vi "MotionCharacterization.vi"() -> ()   [LabVIEW 2011]
panel:
  out "Avg. Motion Time":dbl(knob) scale=0.0..100.0
  out "Joints":T1(graph)
  out "Cartesian":T1(graph)
  out "Coordinates sent to robot:":string
  out "Data Valid?":bool
  out "Motion Timing":u32(graph)
  in  "stop":bool
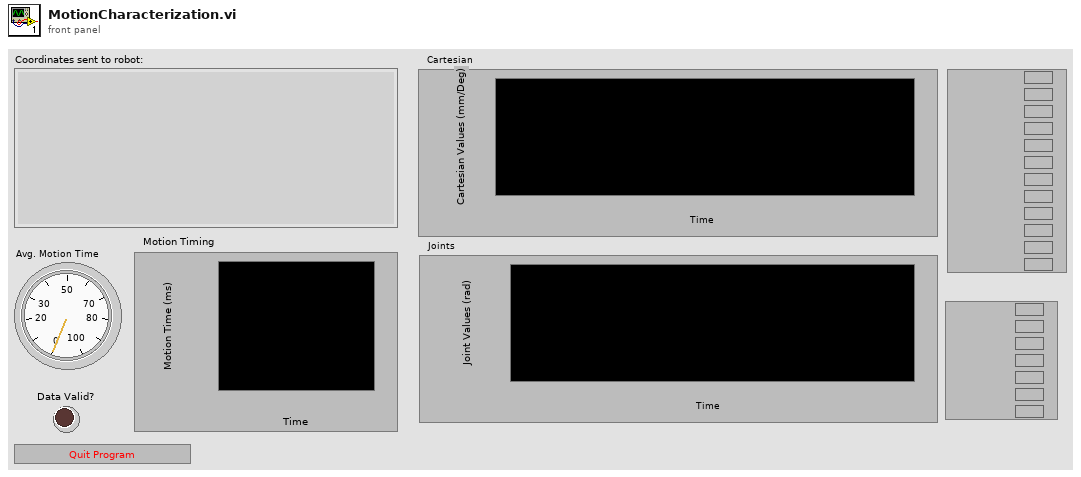
[diagram p1: front panel]
types:
  T1 = cluster{"Data Out[0]":dbl, "Data Out[1]":dbl, "Data Out[2]":dbl, "Data Out[3]":dbl, "Data Out[4]":dbl, "Data Out[5]":dbl, "Data Out[6]":dbl, "Data Out[7]":dbl, "Data Out[8]":dbl}
  T2 = enum16{"Standard", "Buffered", "CRLF", "Immediate"}
  T3 = cluster{"[0]":dbl, "[1]":dbl, "[2]":dbl, "[3]":dbl, "[4]":dbl, "[5]":dbl, "[6]":dbl, "[7]":dbl, "[8]":dbl}
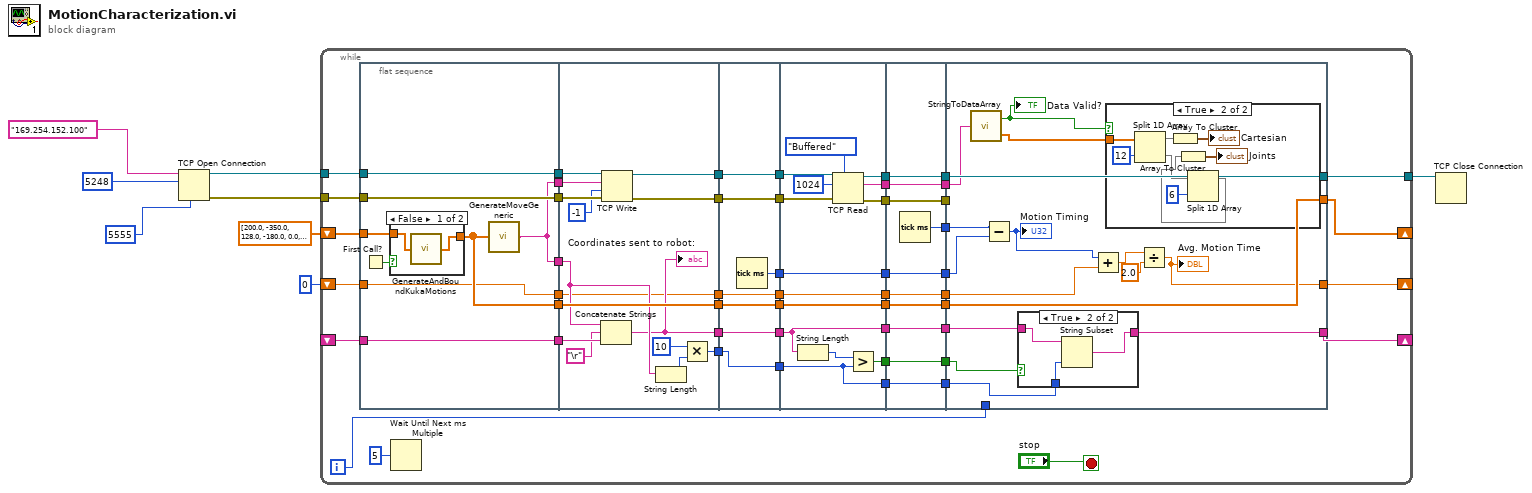
[diagram p0: block diagram]
diagram:
  n1 = TCP Open Connection(address="169.254.152.100", remote port or service name=u16 5248, local port=u16 5555 ("local port (0)")) -> (connection ID=w8:refnum<k5>, error out=w6:errorcluster)  [unwired: 2 in]
  n2 = while {
    tunnel: w8 -> [w58]
    tunnel: [w57] -> w7
    tunnel: w6 -> [w56]
    shift-right: [w37] -> _
    shift-left: dbl[] [200.0, -350.0, 128.0, -180.0, 0.0, 90.0] ("Output Array") -> [w36]
    shift-right: [w26] -> _
    shift-left: _ -> [w28]
    shift-right: [w15] -> _
    shift-left: u32 0 -> [w9]
    i -> [w30]
    stop <- "stop" stop-if-true
    n3 = flat-sequence {
      tunnel: w56 -> [w66]
      tunnel: w58 -> [w67]
      tunnel: [w67] -> w54
      tunnel: [w66] -> w53
      tunnel: [w62] -> w48
      tunnel: w36 -> [w64]
      tunnel: [w63] -> w31
      tunnel: [w62] -> w29
      tunnel: w28 -> [w61]
      tunnel: [w61] -> w27
      tunnel: [w60] -> w10
      tunnel: w9 -> [w60]
      tunnel: [w84] -> w52
      tunnel: [w82] -> w50
      tunnel: w54 -> [w85]
      tunnel: w53 -> [w83]
      tunnel: w48 -> [w81]
      tunnel: [w80] -> w32
      tunnel: w31 -> [w80]
      tunnel: w29 -> [w78]
      tunnel: w27 -> [w77]
      tunnel: [w72] -> w22
      tunnel: [w73] -> w20
      tunnel: [w71] -> w11
      tunnel: w10 -> [w71]
      tunnel: w52 -> [w92]
      tunnel: [w92] -> w51
      tunnel: w50 -> [w91]
      tunnel: [w91] -> w49
      tunnel: [w90] -> w39
      tunnel: [w89] -> w33
      tunnel: w32 -> [w89]
      tunnel: [w88] -> w23
      tunnel: w22 -> [w88]
      tunnel: [w87] -> w21
      tunnel: w20 -> [w87]
      tunnel: [w86] -> w12
      tunnel: w11 -> [w86]
      tunnel: w51 -> [w106]
      tunnel: [w105] -> w47
      tunnel: w49 -> [w104]
      tunnel: [w103] -> w44
      tunnel: [w102] -> w42
      tunnel: [w101] -> w40
      tunnel: w39 -> [w101]
      tunnel: [w100] -> w34
      tunnel: w33 -> [w100]
      tunnel: [w98] -> w24
      tunnel: w23 -> [w98]
      tunnel: w21 -> [w95]
      tunnel: [w96] -> w18
      tunnel: [w95] -> w16
      tunnel: [w93] -> w13
      tunnel: w12 -> [w93]
      tunnel: w47 -> [w116]
      tunnel: [w116] -> w46
      tunnel: [w115] -> w45
      tunnel: w44 -> [w115]
      tunnel: [w108] -> w43
      tunnel: w42 -> [w108]
      tunnel: [w114] -> w41
      tunnel: w40 -> [w114]
      tunnel: [w113] -> w38
      tunnel: [w112] -> w35
      tunnel: w34 -> [w112]
      tunnel: [w111] -> w25
      tunnel: w24 -> [w111]
      tunnel: [w110] -> w19
      tunnel: w18 -> [w110]
      tunnel: [w109] -> w17
      tunnel: w16 -> [w109]
      tunnel: [w107] -> w14
      tunnel: w13 -> [w107]
      tunnel: [w132] -> w57
      tunnel: w46 -> [w132]
      tunnel: w45 -> [_]
      tunnel: w43 -> [w124]
      tunnel: w41 -> [w130]
      tunnel: w38 -> [w131]
      tunnel: [w129] -> w37
      tunnel: w35 -> [w129]
      tunnel: w30 -> [_]
      tunnel: [w126] -> w26
      tunnel: w25 -> [w127]
      tunnel: w19 -> [w128]
      tunnel: w17 -> [w125]
      tunnel: [w117] -> w15
      tunnel: w14 -> [w121]
      frame #0 {
        n4 = First Call?() -> (First Call?: T/F=w65:bool)
        n5 = case shown="False" w65 {
          tunnel: [w68 w70] -> w63
          tunnel: w64 -> [w69 w70]
          frame False {
            n6 = call "GenerateAndBoundKukaMotions.vi"("Output Array"=w69) -> ("Output Array"=w68:dbl[])
          }
          frame True {
          }
        }
        n7 = call "GenerateMoveGeneric.vi"("Input Array"=w63) -> ("Output"=w62:string)
      }
      frame #1 {
        n8 = Concatenate Strings(w78, "\r", w77) -> (w72:string)
        "Coordinates sent to robot:" <- w72
        n9 = TCP Write(connection ID=w85, data in=w81, error in (no error)=w83, 9:-1 ("timeout ms (25000)")) -> (connection ID out=w84:refnum<k5>, error out=w82:errorcluster)  [unwired: 1 out]
        n10 = String Length(string=w78) -> (length=w75:i32)
        n11 = Multiply(x=10, y=w75) -> (x*y=w73:i32)
      }
      frame #2 {
        n12 = Tick Count (ms)() -> (millisecond timer value=w90:u32)
      }
      frame #3 {
        n13 = String Length(string=w98) -> (length=w97:i32)
        n14 = TCP Read(connection ID=w106, bytes to read=1024, error in (no error)=w104, 7:T2."Buffered" ("mode (standard)")) -> (connection ID out=w105:refnum<k5>, data out=w102:string, error out=w103:errorcluster)  [unwired: 1 in]
        n15 = Greater?(x=w97, y=w95) -> (0:w96:bool)
      }
      frame #4 {
        n16 = Tick Count (ms)() -> (millisecond timer value=w113:u32)
      }
      frame #5 {
        n17 = call "StringToDataArray.vi"("Data In"=w124) -> ("Good Data"=w122:bool, "Data Out"=w123:dbl[])
        "Data Valid?" <- w122
        n18 = Subtract(x=w131, y=w130) -> (x-y=w120:u32)
        "Motion Timing" <- w120
        n19 = case shown="True" w128 {
          tunnel: w127 -> [w141 w144]
          tunnel: [w141 w142] -> w126
          tunnel: w125 -> [_ w143]
          frame False {
          }
          frame True {
            n20 = String Subset(string=w144, length (rest)=w143) -> (substring=w142:string)  [unwired: 1 in]
          }
        }
        n21 = Add(x=w120, y=w121) -> (x+y=w118:dbl)
        n22 = case shown="True" w122 {
          tunnel: w123 -> [_ w139]
          frame False {
          }
          frame True {
            n23 = Split 1D Array(array=w139, index=12) -> (first subarray=w136:dbl[], second subarray=w135:dbl[])
            n24 = Array To Cluster(array=w136) -> (cluster=→"Cartesian":T3)
            n25 = Split 1D Array(array=w135, index=6) -> (first subarray=w133:dbl[])  [unwired: 1 out]
            n26 = Array To Cluster(array=w133) -> (cluster=→"Joints":T3)
          }
        }
        n27 = Divide(x=w118, y=2.0) -> (x/y=w117:dbl)
        "Avg. Motion Time" <- w117
      }
    }
    n28 = Wait Until Next ms Multiple(millisecond multiple=u32 5) -> ()  [unwired: 1 out]
  }
  n29 = TCP Close Connection(connection ID=w7) -> ()  [unwired: 2 in, 2 out]
